vi "[SubV]PDControlRight.vi"(6 "PV Old":fxp<+/-,64,32>, 8 "Kd":fxp<+/-,64,32>, 9 "Kp":fxp<+/-,64,32>, 10 "PV":fxp<+/-,64,32>, 11 "SP":fxp<+/-,64,32>) -> (2 "PV Out":fxp<+/-,64,32>, 3 "Right Out":fxp<+/-,64,32>)   [LabVIEW 2019]
uses:
  <vilib>/rvi/Emulation/niFpgaGetClockAttributes.vi
  <vilib>/rvi/Emulation/niFpgaSctlEmulationGetInTimedLoop.vi
  <vilib>/rvi/Emulation/niFpgaEmulationReportErrorSimple.vi
  <vilib>/rvi/Emulation/niFpgaCriticalErrorInLSC.vi
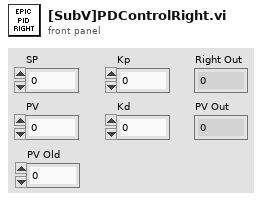
[diagram p1: front panel]
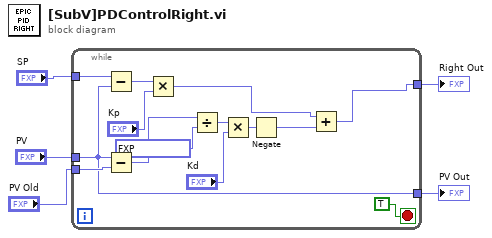
[diagram p0: block diagram]
diagram:
  n1 = while {
    tunnel: "SP" -> [w18]
    tunnel: "PV" -> [w9]
    tunnel: [w6] -> w4
    tunnel: "PV Old" -> [w16]
    tunnel: [w9] -> w1
    stop <- TRUE ("stop") stop-if-true
    n2 = Subtract(x=w18, y=w9) -> (x-y=w11:fxp<+/-,64,33>)
    n3 = Subtract(x=w9, y=w16) -> (x-y=w15:fxp<+/-,64,33>)
    n4 = Multiply(x=w11, y="Kp") -> (x*y=w7:fxp<+/-,64,65>)
    n5 = Divide(x=w15, y=fxp<+,5,-9> 0.0009765625) -> (x/y=w13:fxp<+/-,64,44>)
    n6 = Multiply(x=w13, y="Kd") -> (x*y=w10:fxp<+/-,64,76>)
    n7 = Negate(x=w10) -> (-x=w8:fxp<+/-,64,77>)
    n8 = Add(x=w7, y=w8) -> (x+y=w6:fxp<+/-,64,78>)
  }
  "Right Out" <- w4
  "PV Out" <- w1
